vi "Room to Hallway.vi"(11 "State in":cluster{"Hallway":string[], "Rooms":string[][]}) -> (2 "Best Cost":u64, 3 "State out":cluster{"Hallway":string[], "Rooms":string[][]})   [LabVIEW 2019, in "23.lvlib"]
uses:
  23.lvlib
  Between.vi
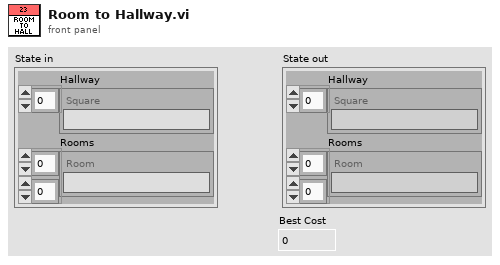
[diagram p1: front panel]
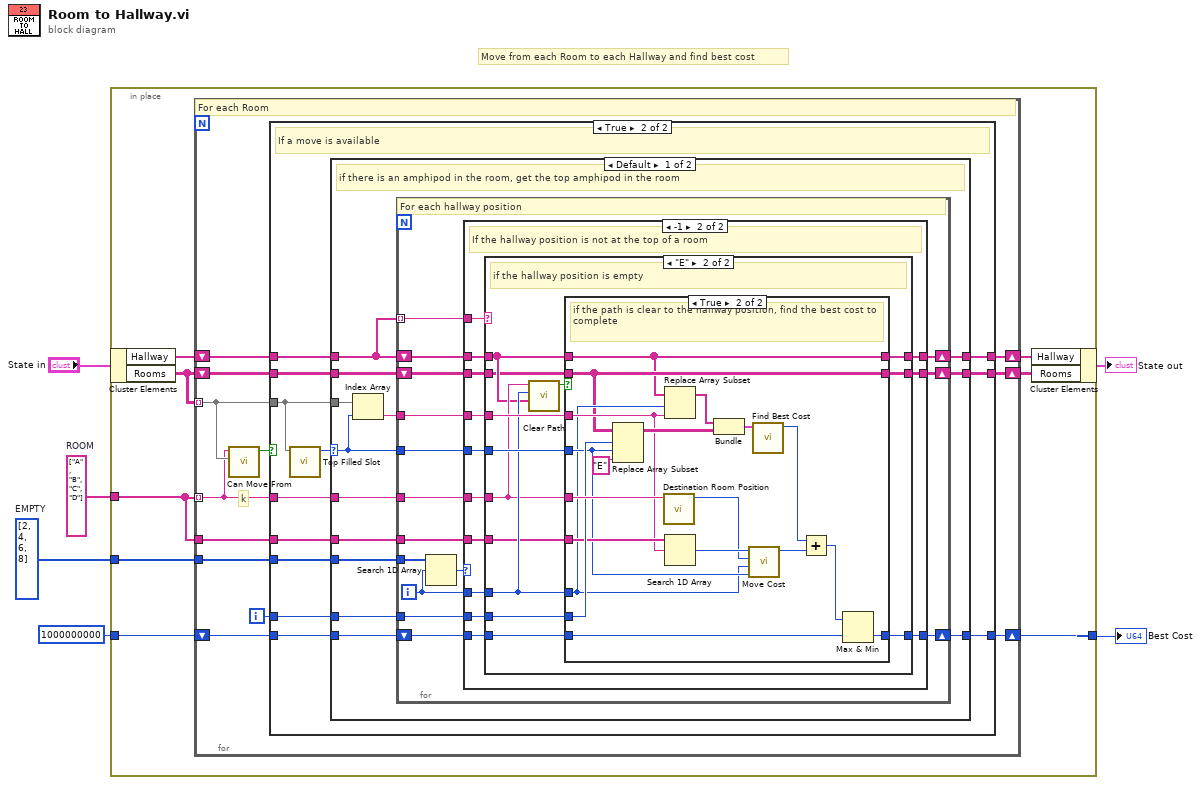
[diagram p0: block diagram]
diagram:
  w2 = string[] ["A", "B", "C", "D"]  # ROOM
  w4 = u64[] [2, 4, 6, 8]  # EMPTY
  # "Move from each Room to each Hallway and find best cost"
  n1 = in-place {
    in-place-border: [w14] -> w6
    in-place-border: w4 -> [w11]
    in-place-border: u64 1000000000 ("Best Cost") -> [w10]
    in-place-border: w2 -> [w9]
    n2 = in-place-cluster #1("State in") -> ("Hallway"=w13:string[], "Rooms"=w12:string[][])
    n3 = for {
      tunnel: w12 -> [w25] mode=indexing
      tunnel: w9 -> [w23] mode=indexing
      shift-right: [w19] -> w14
      shift-left: w10 -> [w20]
      tunnel: w11 -> [w18]
      tunnel: w9 -> [w17]
      shift-right: [w15] -> w8
      shift-left: w13 -> [w24]
      shift-right: [w16] -> w7
      shift-left: w12 -> [w22]
      i -> [w21]
      # "k"
      # "For each Room"
      n4 = call "Can Move From.vi"("Room"=w25, "Amphipod"=w23) -> ("Can Move From?"=w26:bool)  [unwired: 9 in]
      n5 = case shown="True" w26 {
        tunnel: w25 -> [_ w40]
        tunnel: w24 -> [w28 w39]
        tunnel: w18 -> [_ w38]
        tunnel: w23 -> [_ w37]
        tunnel: w22 -> [w27 w36]
        tunnel: w21 -> [_ w35]
        tunnel: w17 -> [_ w34]
        tunnel: w20 -> [w29 w33]
        tunnel: [w29 w32] -> w19
        tunnel: [w27 w31] -> w16
        tunnel: [w28 w30] -> w15
        frame False {
          # "If a move is not available try the next room"
        }
        frame True {
          # "If a move is available"
          n6 = call "Top Filled Slot.vi"("Room"=w40) -> ("Top Filled Slot"=w41:i32)  [unwired: 10 in]
          n7 = case shown="Default" w41 {
            selector: w41 -> [w51 _]
            tunnel: w40 -> [w49 _]
            tunnel: w39 -> [w52 w125]
            tunnel: w38 -> [w54 _]
            tunnel: w37 -> [w53 _]
            tunnel: w36 -> [w48 w124]
            tunnel: w35 -> [w47 _]
            tunnel: w34 -> [w46 _]
            tunnel: w33 -> [w45 w126]
            tunnel: [w44 w126] -> w32
            tunnel: [w43 w124] -> w31
            tunnel: [w42 w125] -> w30
            frame Default {
              # "if there is an amphipod in the room, get the top amphipod in the room"
              n8 = Index Array(array=w49, index=w51) -> (element=w50:string)
              n9 = for {
                tunnel: w52 -> [w67] mode=indexing
                tunnel: w54 -> [w69]
                tunnel: w53 -> [w66]
                tunnel: w51 -> [w63]
                tunnel: w50 -> [w62]
                tunnel: w47 -> [w60]
                tunnel: w46 -> [w59]
                shift-right: [w57] -> w44
                shift-left: w45 -> [w58]
                shift-right: [w56] -> w43
                shift-left: w48 -> [w61]
                shift-right: [w55] -> w42
                shift-left: w52 -> [w64]
                i -> [w65]
                # "For each hallway position"
                n10 = Search 1D Array(1D array=w69, element=w65) -> (index of element=w68:i32)  [unwired: 1 in]
                n11 = case shown="-1" w68 {
                  tunnel: w67 -> [_ w85]
                  tunnel: w66 -> [_ w84]
                  tunnel: w65 -> [_ w83]
                  tunnel: w64 -> [w71 w82]
                  tunnel: w63 -> [_ w81]
                  tunnel: w62 -> [_ w80]
                  tunnel: w61 -> [w70 w79]
                  tunnel: w60 -> [_ w78]
                  tunnel: w59 -> [_ w77]
                  tunnel: w58 -> [w72 w76]
                  tunnel: [w72 w75] -> w57
                  tunnel: [w70 w74] -> w56
                  tunnel: [w71 w73] -> w55
                  frame Default {
                    # "if the hallway position is at the top of a room try the next one"
                  }
                  frame -1 {
                    # "If the hallway position is not at the top of a room"
                    n12 = case shown="\"E\"" w85 {
                      tunnel: w84 -> [_ w97]
                      tunnel: w83 -> [_ w98]
                      tunnel: w82 -> [w87 w96]
                      tunnel: w81 -> [_ w100]
                      tunnel: w80 -> [_ w99]
                      tunnel: w79 -> [w86 w95]
                      tunnel: w78 -> [_ w94]
                      tunnel: w77 -> [_ w93]
                      tunnel: w76 -> [w88 w92]
                      tunnel: [w88 w91] -> w75
                      tunnel: [w86 w90] -> w74
                      tunnel: [w87 w89] -> w73
                      frame Default {
                        # "if the hallway position is filled, try the next one"
                      }
                      frame "E" {
                        # "if the hallway position is empty"
                        n13 = call "Clear Path.vi"("Hallway"=w96, "Hallway Position"=w98, "Room"=w97) -> ("Clear Path?"=w101:bool)  [unwired: 8 in]
                        n14 = case shown="True" w101 {
                          tunnel: w100 -> [_ w110]
                          tunnel: w99 -> [_ w112]
                          tunnel: w98 -> [_ w108]
                          tunnel: w97 -> [_ w123]
                          tunnel: w96 -> [w103 w105]
                          tunnel: w95 -> [w102 w106]
                          tunnel: w94 -> [_ w119]
                          tunnel: w93 -> [_ w117]
                          tunnel: w92 -> [w104 w114]
                          tunnel: [w104 w113] -> w91
                          tunnel: [w102 w106] -> w90
                          tunnel: [w103 w105] -> w89
                          frame False {
                          }
                          frame True {
                            # "if the path is clear to the hallway position, find the best cost to complete"
                            n15 = Replace Array Subset(array=w106, new element="E" ("y"), index (row)=w119, index (col)=w110) -> (w120:string[][])
                            n16 = call "Destination Room Position.vi"("Amphipod Type"=w123) -> ("Destination Room Position"=w109:i32)  [unwired: 10 in]
                            n17 = Replace Array Subset(array=w105, new element=w112, index=w108) -> (w122:string[])
                            n18 = Search 1D Array(1D array=w117, element=w112) -> (index of element=w111:i32)  [unwired: 1 in]
                            n19 = Bundle("Hallway"=w122, "Rooms"=w120) -> (w121:cluster{"Hallway":string[], "Rooms":string[][]})  [unwired: 1 in]
                            n20 = call "Move Cost.vi"("Room Slot"=w110, "Destination Position"=w108, "Source Position"=w109, "Amphipod Type Index"=w111) -> ("Move Cost"=w107:u64)  [unwired: 7 in]
                            n21 = call "Find Best Cost.vi"("State"=w121) -> ("Best Cost"=w116:u64)  [unwired: 10 in]
                            n22 = Add(x=w116, y=w107) -> (x+y=w115:u64)
                            n23 = Max & Min(x=w115, y=w114) -> (min(x,y)=w113:u64)  [unwired: 1 out]
                          }
                        }
                      }
                    }
                  }
                }
              }
            }
            frame -1 {
              # "if there is no amphipod in the room, try the next one"
            }
          }
        }
      }
    }
    n24 = in-place-cluster #1("Hallway"=w8, "Rooms"=w7) -> (→"State out":cluster{"Hallway":string[], "Rooms":string[][]})
  }
  "Best Cost" <- w6
